vi "Temperatura_Y_Pinzas.vi"() -> ()   [LabVIEW 2010]
uses:
  <vilib>/express/express analysis/Spectral/XNode/ExpressSpectralMeasurementsBlockNode.xnode
  <vilib>/express/express analysis/Spectral/Block/exnSpectralBlock spectral measurements RMS poly.vi
  <vilib>/express/express analysis/Spectral/Block/exnSpectralBlock spectral measurements RMS DDT.vi
panel:
  out "Pinza 5":dynamicdata(graph)
  out "Pinza 4":dbl format="%#_5g"
  out "Verde":dbl format="%#_5g"
  out "Pinza 3":dynamicdata(graph)
  out "Pinza 3":dbl format="%#_5g"
  out "Morada":dbl format="%#_5g"
  out "Pinza 2":dynamicdata(graph)
  out "Pinza 2":dbl format="%#_5g"
  out "Azul":dbl format="%#_5g"
  in  "stop 3":bool
  out "Pinza":dynamicdata(graph)
  out "Waveform Graph 3":dynamicdata(graph)
  out "Termocupla":dbl format="%#.4g"
  out "Pinza":dbl format="%#_5g"
  out "Waveform Graph 2":dynamicdata(graph)
  out "Rosada":dbl format="%#_5g"
  in  "stop":bool
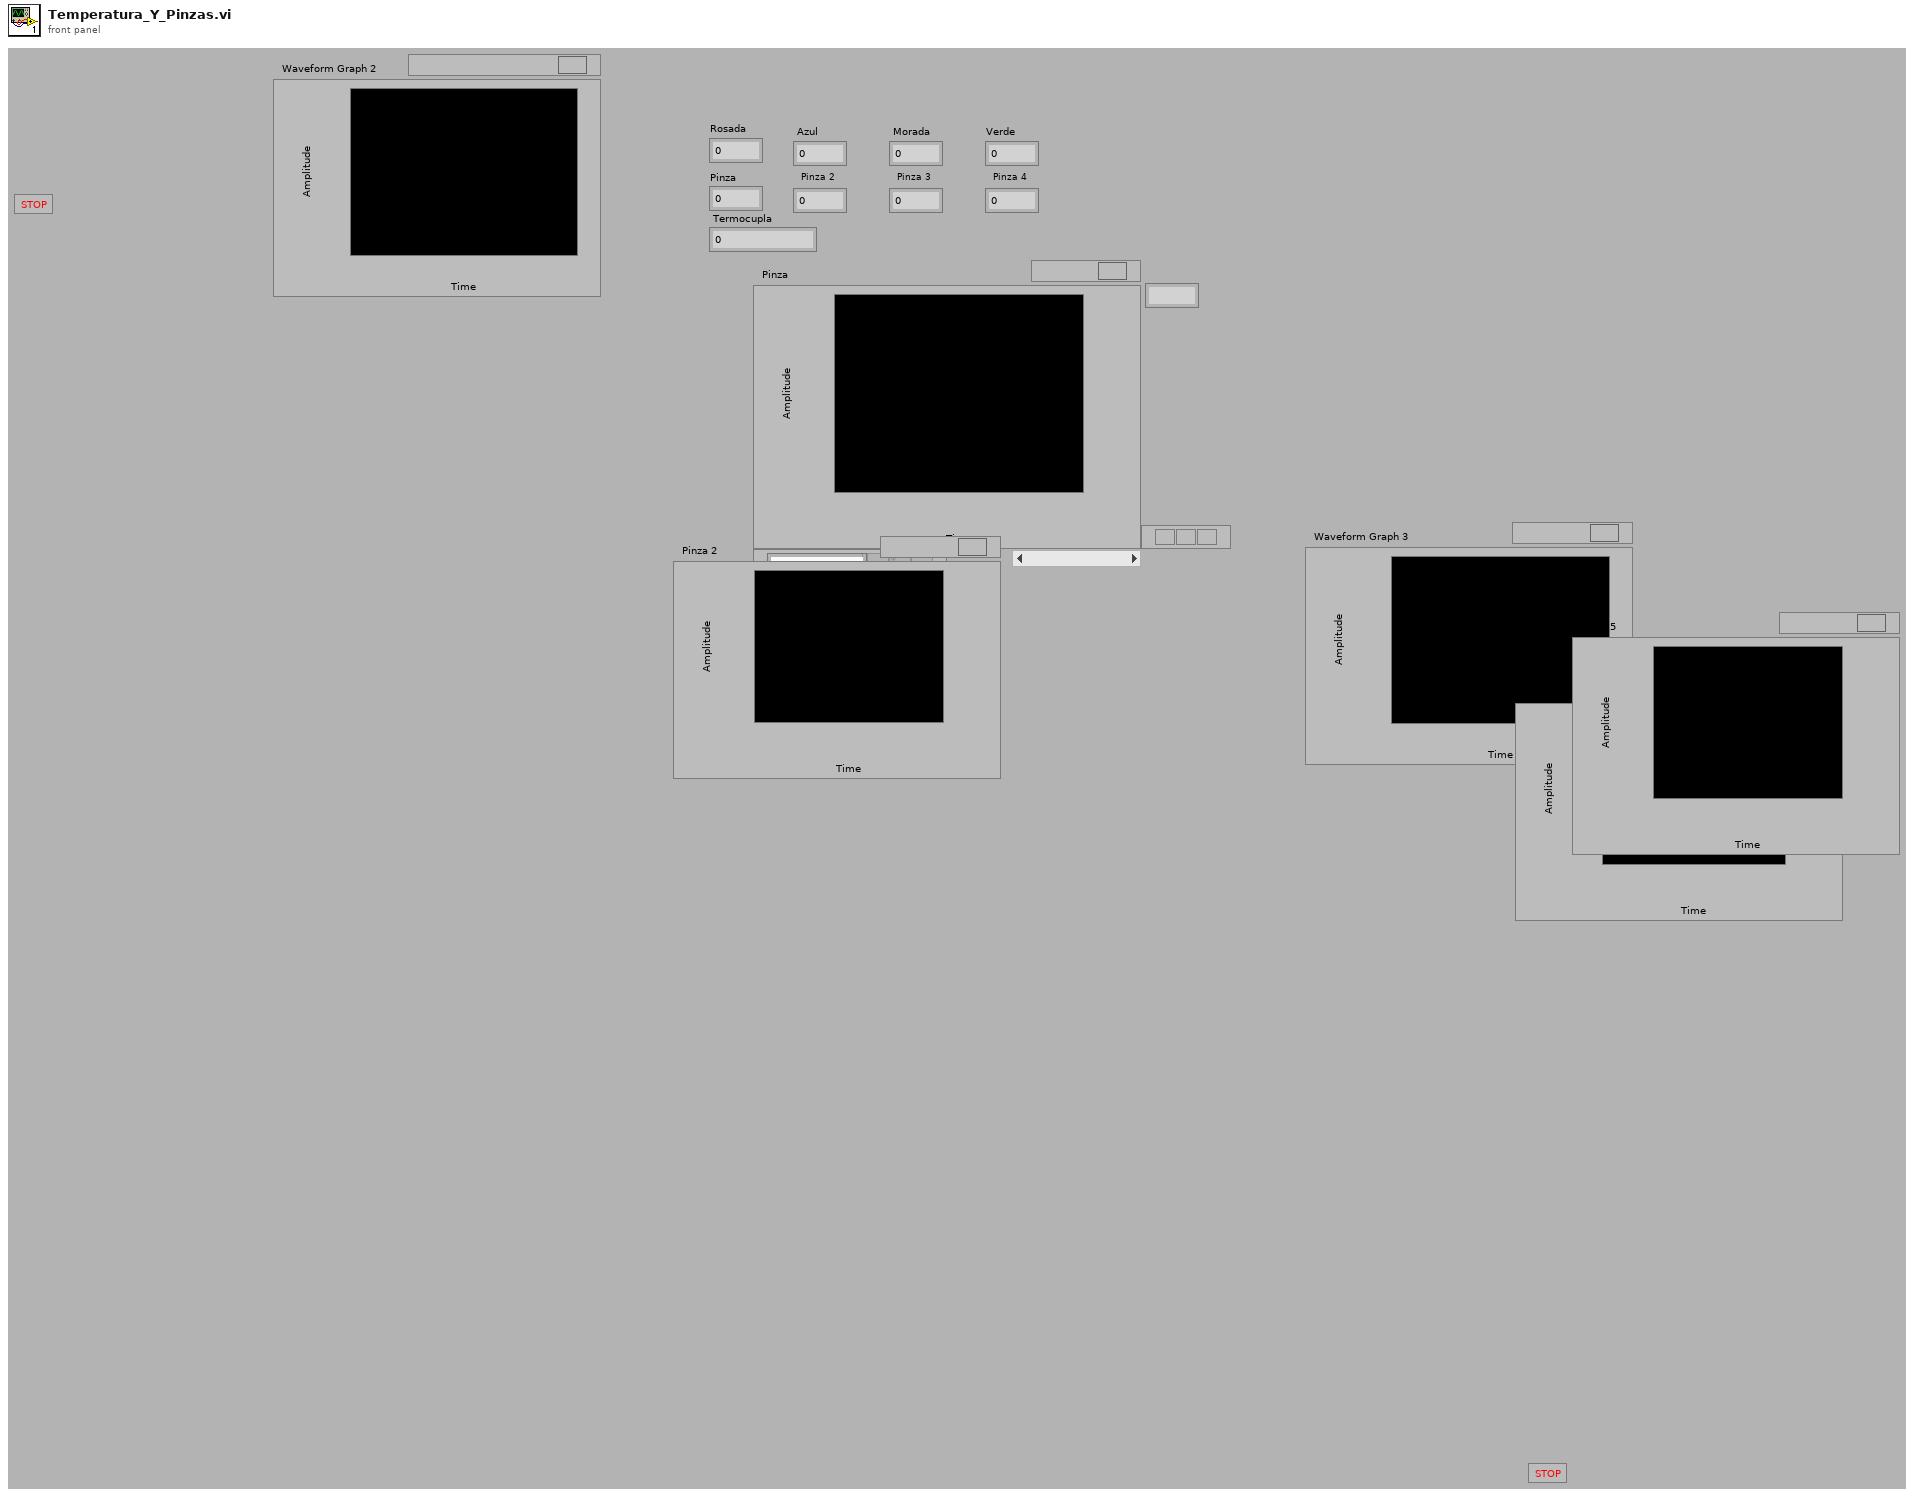
[diagram p1: front panel]
types:
  T1 = cluster{"averaging mode":u16, "weighting mode":u16, "number of averages":u32}
  T2 = cluster{"dB On (F)":bool, "unwrap phase (F)":bool, "convert to degree (F)":bool}
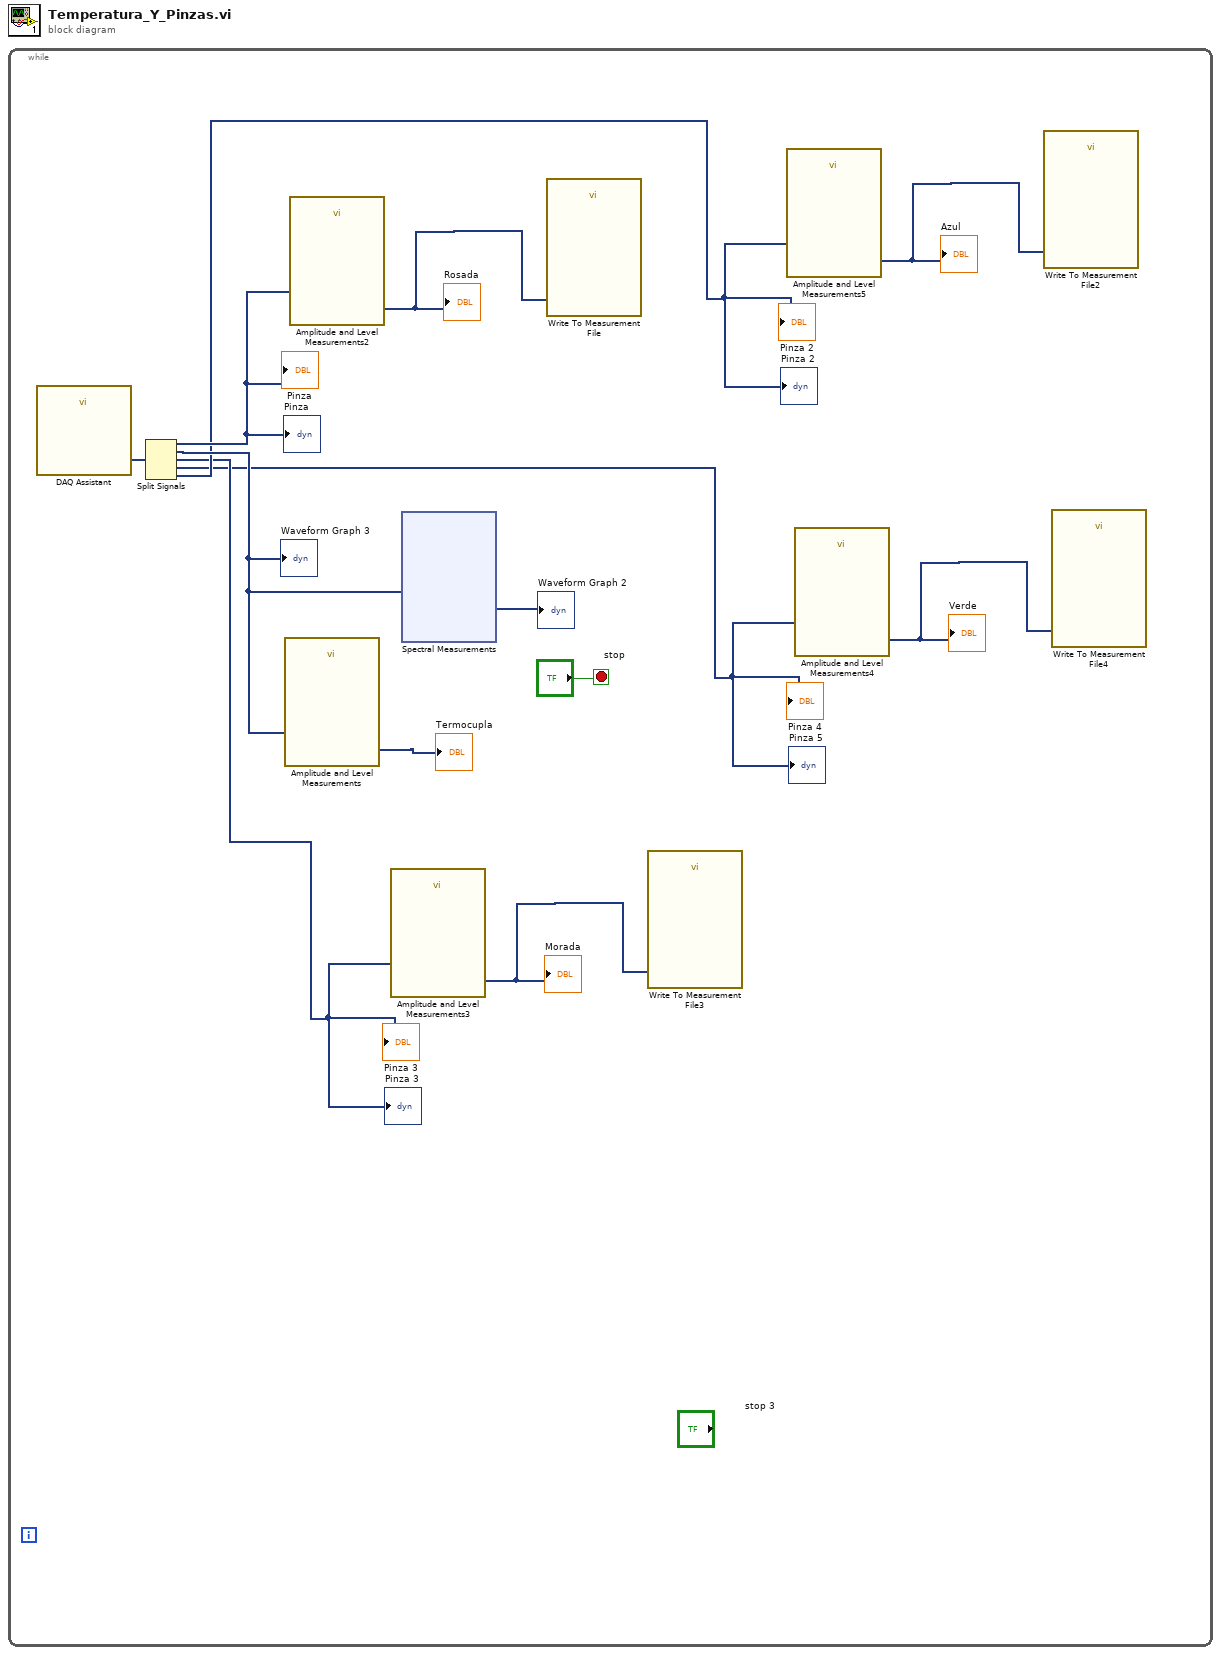
[diagram p0: block diagram]
diagram:
  n1 = while {
    stop <- "stop" stop-if-true
    n2 = call "DAQ Assistant"() -> ("data"=w11:dynamicdata)  [unwired: 16 in, 3 out]
    n3 = Split Signals(w11) -> (w8:dynamicdata, w9:dynamicdata, w3:dynamicdata, w1:dynamicdata, w5:dynamicdata)  [unwired: 5 in]
    "Pinza" <- w8
    "Waveform Graph 3" <- w9
    "Pinza" <- w8
    "Pinza 2" <- w5
    "Pinza 2" <- w5
    "Pinza 3" <- w3
    "Pinza 3" <- w3
    "Pinza 4" <- w1
    "Pinza 5" <- w1
    n4 = call "Amplitude and Level Measurements"("Signals"=w9) -> ("Mean (DC)"=→"Termocupla":dynamicdata)  [unwired: 13 in, 1 out]
    n5 = call "Amplitude and Level Measurements2"("Signals"=w8) -> ("Mean (DC)"=w12:dynamicdata)  [unwired: 13 in, 1 out]
    "Rosada" <- w12
    n6 = call "Amplitude and Level Measurements3"("Signals"=w3) -> ("Mean (DC)"=w4:dynamicdata)  [unwired: 13 in, 1 out]
    "Morada" <- w4
    n7 = xnode "Spectral Measurements"("Signals"=w9) -> ("FFT - (RMS)"=→"Waveform Graph 2":dynamicdata)  [unwired: 1 in, 2 out]
    n8 = call "Write To Measurement File"("Signals"=w12) -> ()  [unwired: 16 in, 3 out]
    n9 = call "Write To Measurement File3"("Signals"=w4) -> ()  [unwired: 16 in, 3 out]
    n10 = call "Amplitude and Level Measurements5"("Signals"=w5) -> ("Mean (DC)"=w6:dynamicdata)  [unwired: 13 in, 1 out]
    "Azul" <- w6
    n11 = call "Amplitude and Level Measurements4"("Signals"=w1) -> ("Mean (DC)"=w2:dynamicdata)  [unwired: 13 in, 1 out]
    "Verde" <- w2
    n12 = call "Write To Measurement File2"("Signals"=w6) -> ()  [unwired: 16 in, 3 out]
    n13 = call "Write To Measurement File4"("Signals"=w2) -> ()  [unwired: 16 in, 3 out]
  }
